vi "SCLN_ReleaseServers.vi"(5 "Server Name":string) -> ()   [LabVIEW 2015]
doc: "Function : Load with initial values globals type II.\n\n It loads with necessary initial values some variables\n type II, which are used during the execution of the program.\n \nInput Parameters: \n\n None.\n\nOutput Parameters:\n\n None."
uses:
  SCLN_RW_Select.ctl
  SCLN_INT32_Select.ctl
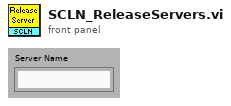
[diagram p1: front panel]
types:
  T1 = typedef "SCLN_INT32_Select.ctl" = enum16{"Max_Servers", "Max_Clients", "Total_Servers", "Total_Clients"}
  T2 = typedef "SCLN_RW_Select.ctl" = enum16{"Read", "Write"}
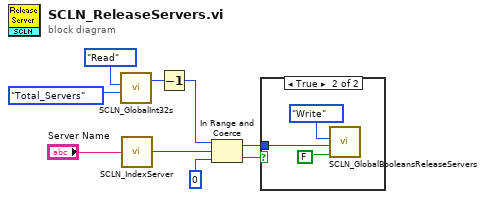
[diagram p0: block diagram]
diagram:
  n1 = call "SCLN_GlobalInt32s.vi"("Element"=SCLN_INT32_Select."Total_Servers" ("GBL_INT32"), "Operation"=SCLN_RW_Select."Read" ("GBL_RW")) -> ("Read Value"=w2:i32)  [unwired: 2 in, 1 out]
  n2 = call "SCLN_IndexServer.vi"("Server Name"="Server Name") -> ("Index"=w7:i32)
  n3 = Decrement(x=w2) -> (x-1=w1:i32)
  n4 = In Range and Coerce(upper limit=w1, x=w7, lower limit=0) -> (coerced(x)=w5:i32, In Range?=w6:bool)
  n5 = case shown="True" w6 {
    tunnel: w5 -> [_ w10]
    frame False {
    }
    frame True {
      n6 = call "SCLN_GlobalBooleansReleaseServers.vi"("Write Value"=FALSE, "Element"=w10, "Operation"=SCLN_RW_Select."Write" ("GBL_RW")) -> ()  [unwired: 1 in, 2 out]
    }
  }
